vi "CalSumv.vi"(0 "AD1":u64, 1 "AD2":u64, 2 "REAL1":dbl, 3 "REAL2":dbl, 5 "InOrOut":u16(ring) items=["InSumv"=2, "OutSumv"=3], 8 "类型":u32(ring)=4 items=["PCI5121"=1, "PCI9810"=2, "USBCAN1"=3, "USBCAN2"=4, "PCI9820"=5, "CAN232"=6, "PCI5110"=7, "CANLite(mini)"=8, "ISA9620"=9, "ISA5420"=10, "PC104CAN"=11, "CANET"=17, "DNP9810"=13, "USBCAN-E-U"=20, "USBCAN-2E-U"=21], 10 "设备索引":u32(ring) items=["0", "1", "2", "3", "4", "5", "6", "7", "8", "9", "10", "11", "12", "13", "14", "15", ""], 12 "CAN路数":u32(ring) items=["0", "1"], 14 "ExternFlag":u8, 16 "ID Send":u32, 18 "DataLen":u8) -> (20 "发送状态":bool, 21 "Gain":dbl, 22 "Offset":i32 format="%x")   [LabVIEW 2013]
uses:
  BHN01/AutoBurn/Settings/ControlCAN.dll
panel:
  in  "设备索引 2":u32(ring) items=["0", "1", "2", "3", "4", "5", "6", "7", "8", "9", "10", "11", "12", "13", "14", "15", ""]
  in  "CAN路数 2":u32(ring) items=["0", "1"]
  in  "类型 2":u32(ring)=4 items=["PCI5121"=1, "PCI9810"=2, "USBCAN1"=3, "USBCAN2"=4, "PCI9820"=5, "CAN232"=6, "PCI5110"=7, "CANLite(mini)"=8, "ISA9620"=9, "ISA5420"=10, "PC104CAN"=11, "CANET"=17, "DNP9810"=13, "USBCAN-E-U"=20, "USBCAN-2E-U"=21]
  out "VCI_CAN_OBJ_T":T1 {"ID" format="%x"}
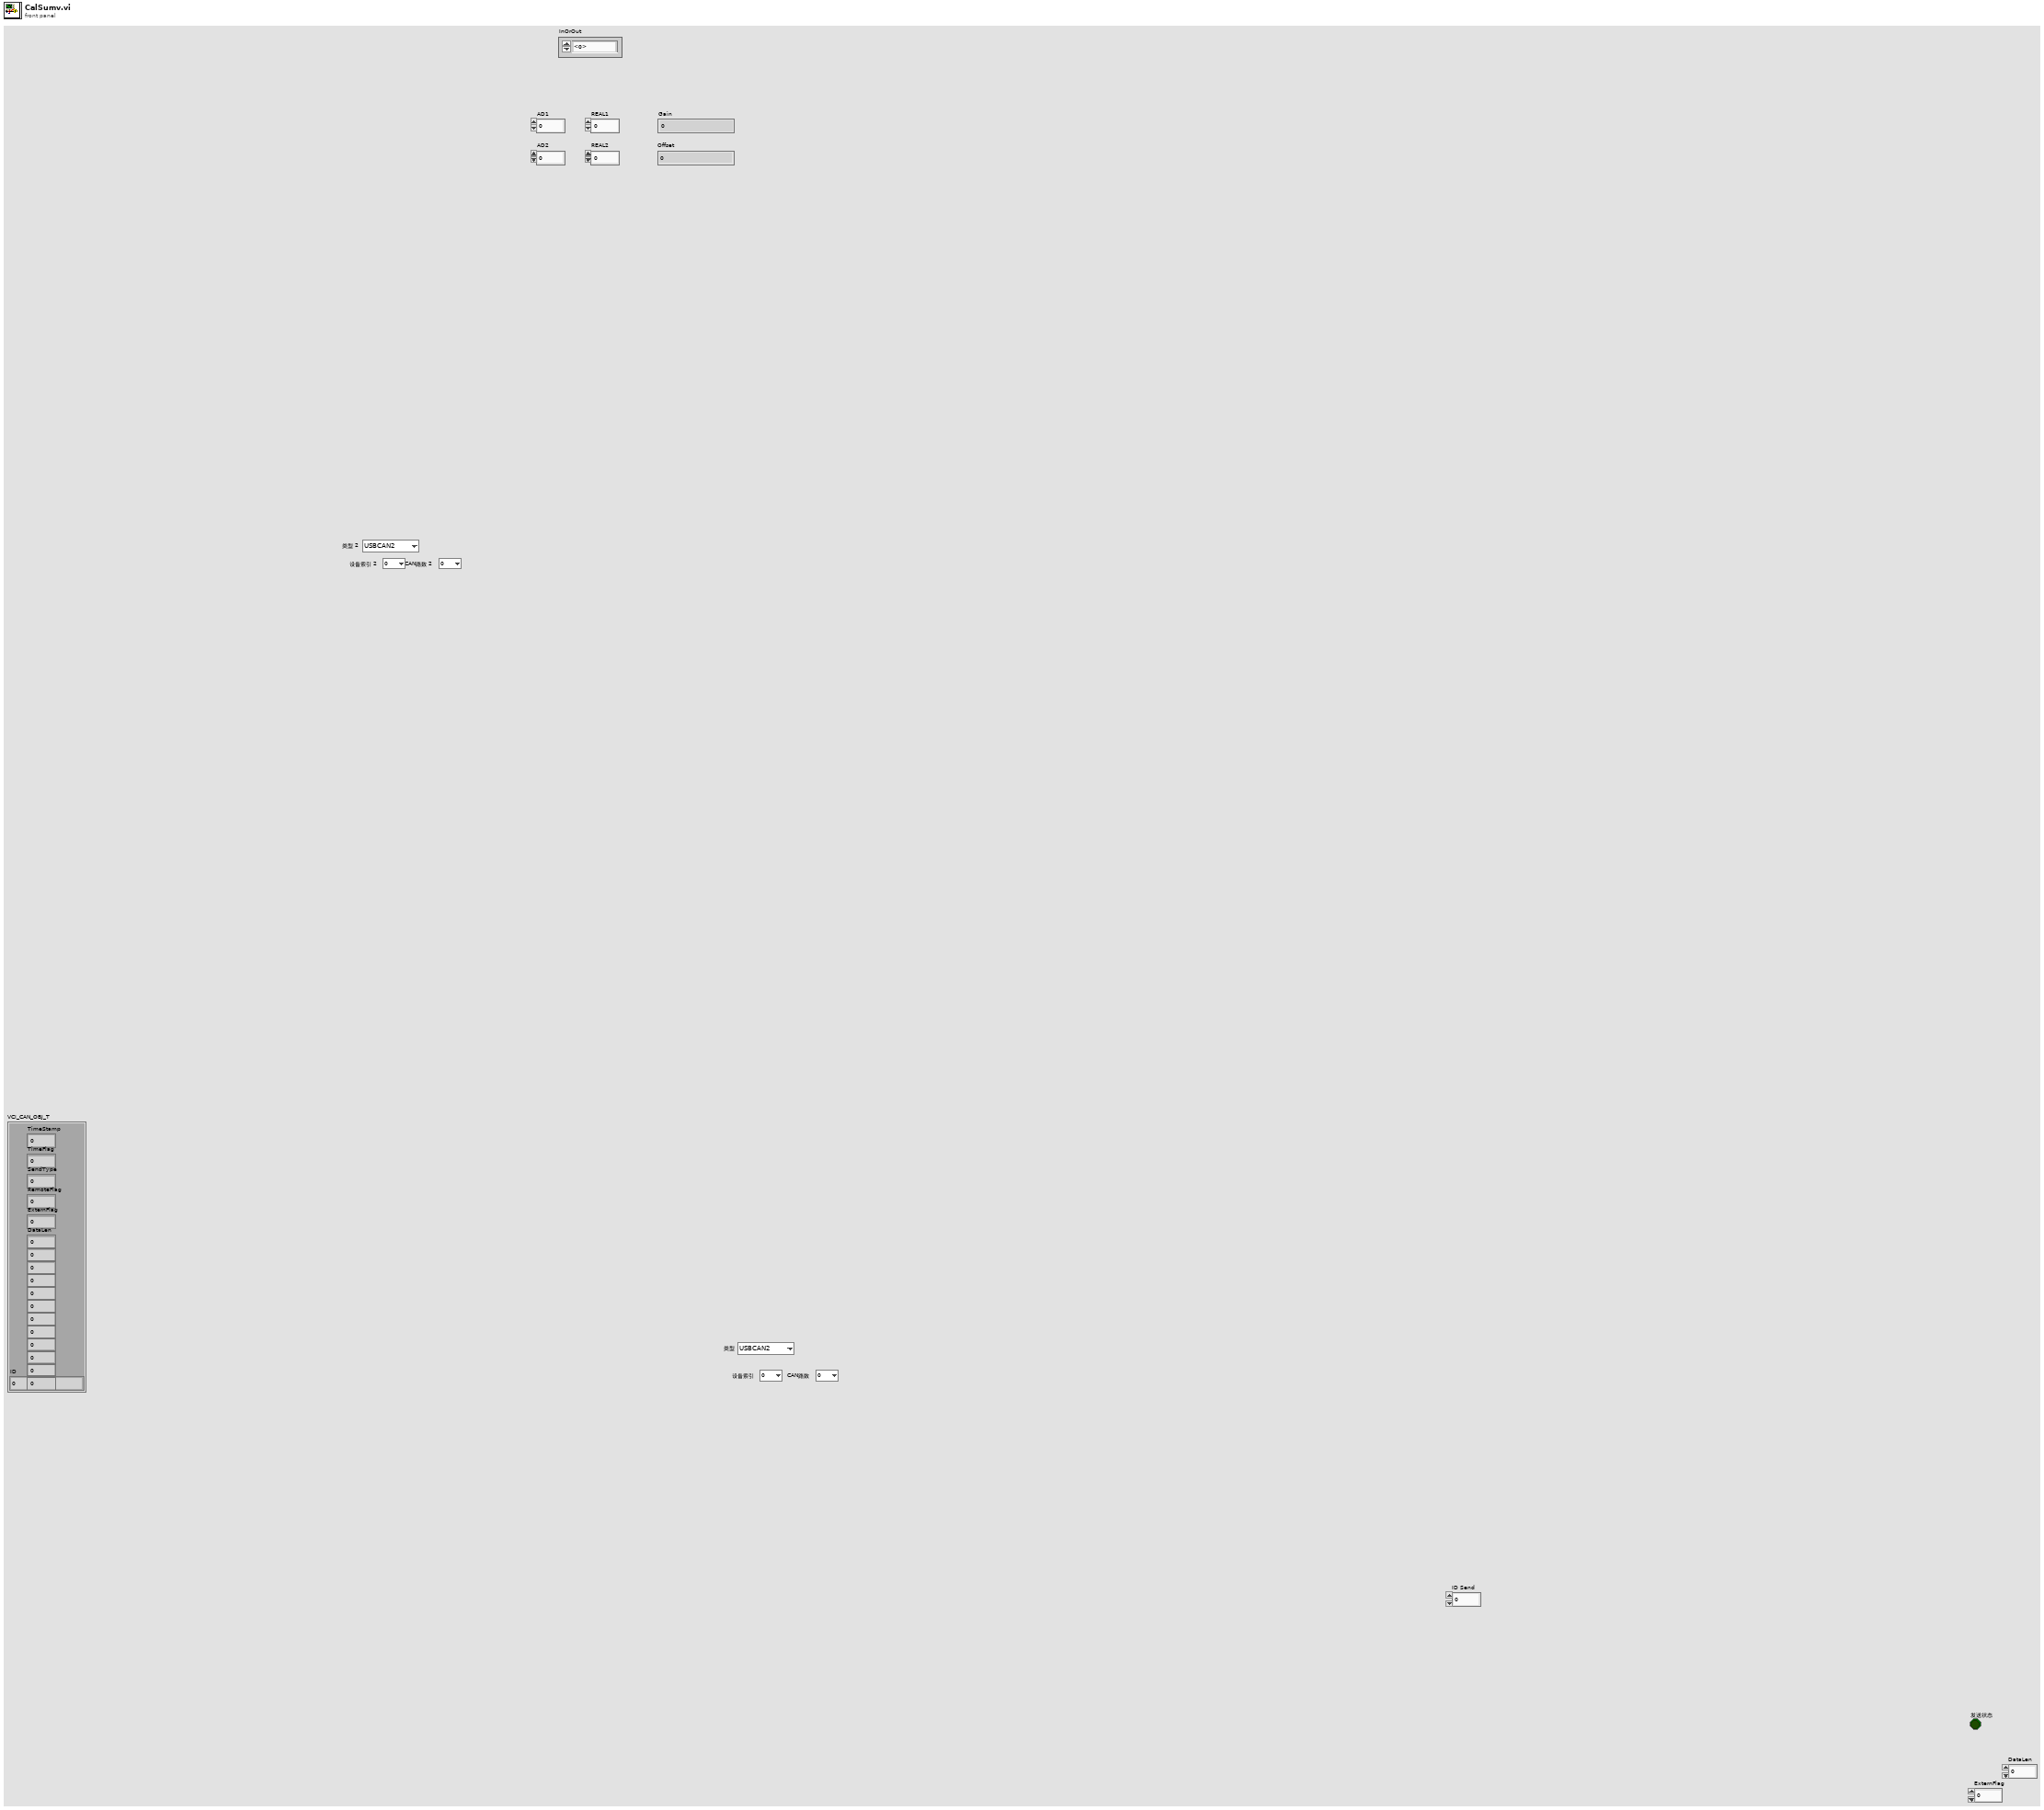
[diagram p1: front panel]
types:
  T1 = cluster{"ID":u32, "TimeStamp":u32, "TimeFlag":u8, "SendType":u8, "RemoteFlag":u8, "ExternFlag":u8, "DataLen":u8, u8, u8, u8, u8, u8, u8, u8, u8, u8, u8, u8}
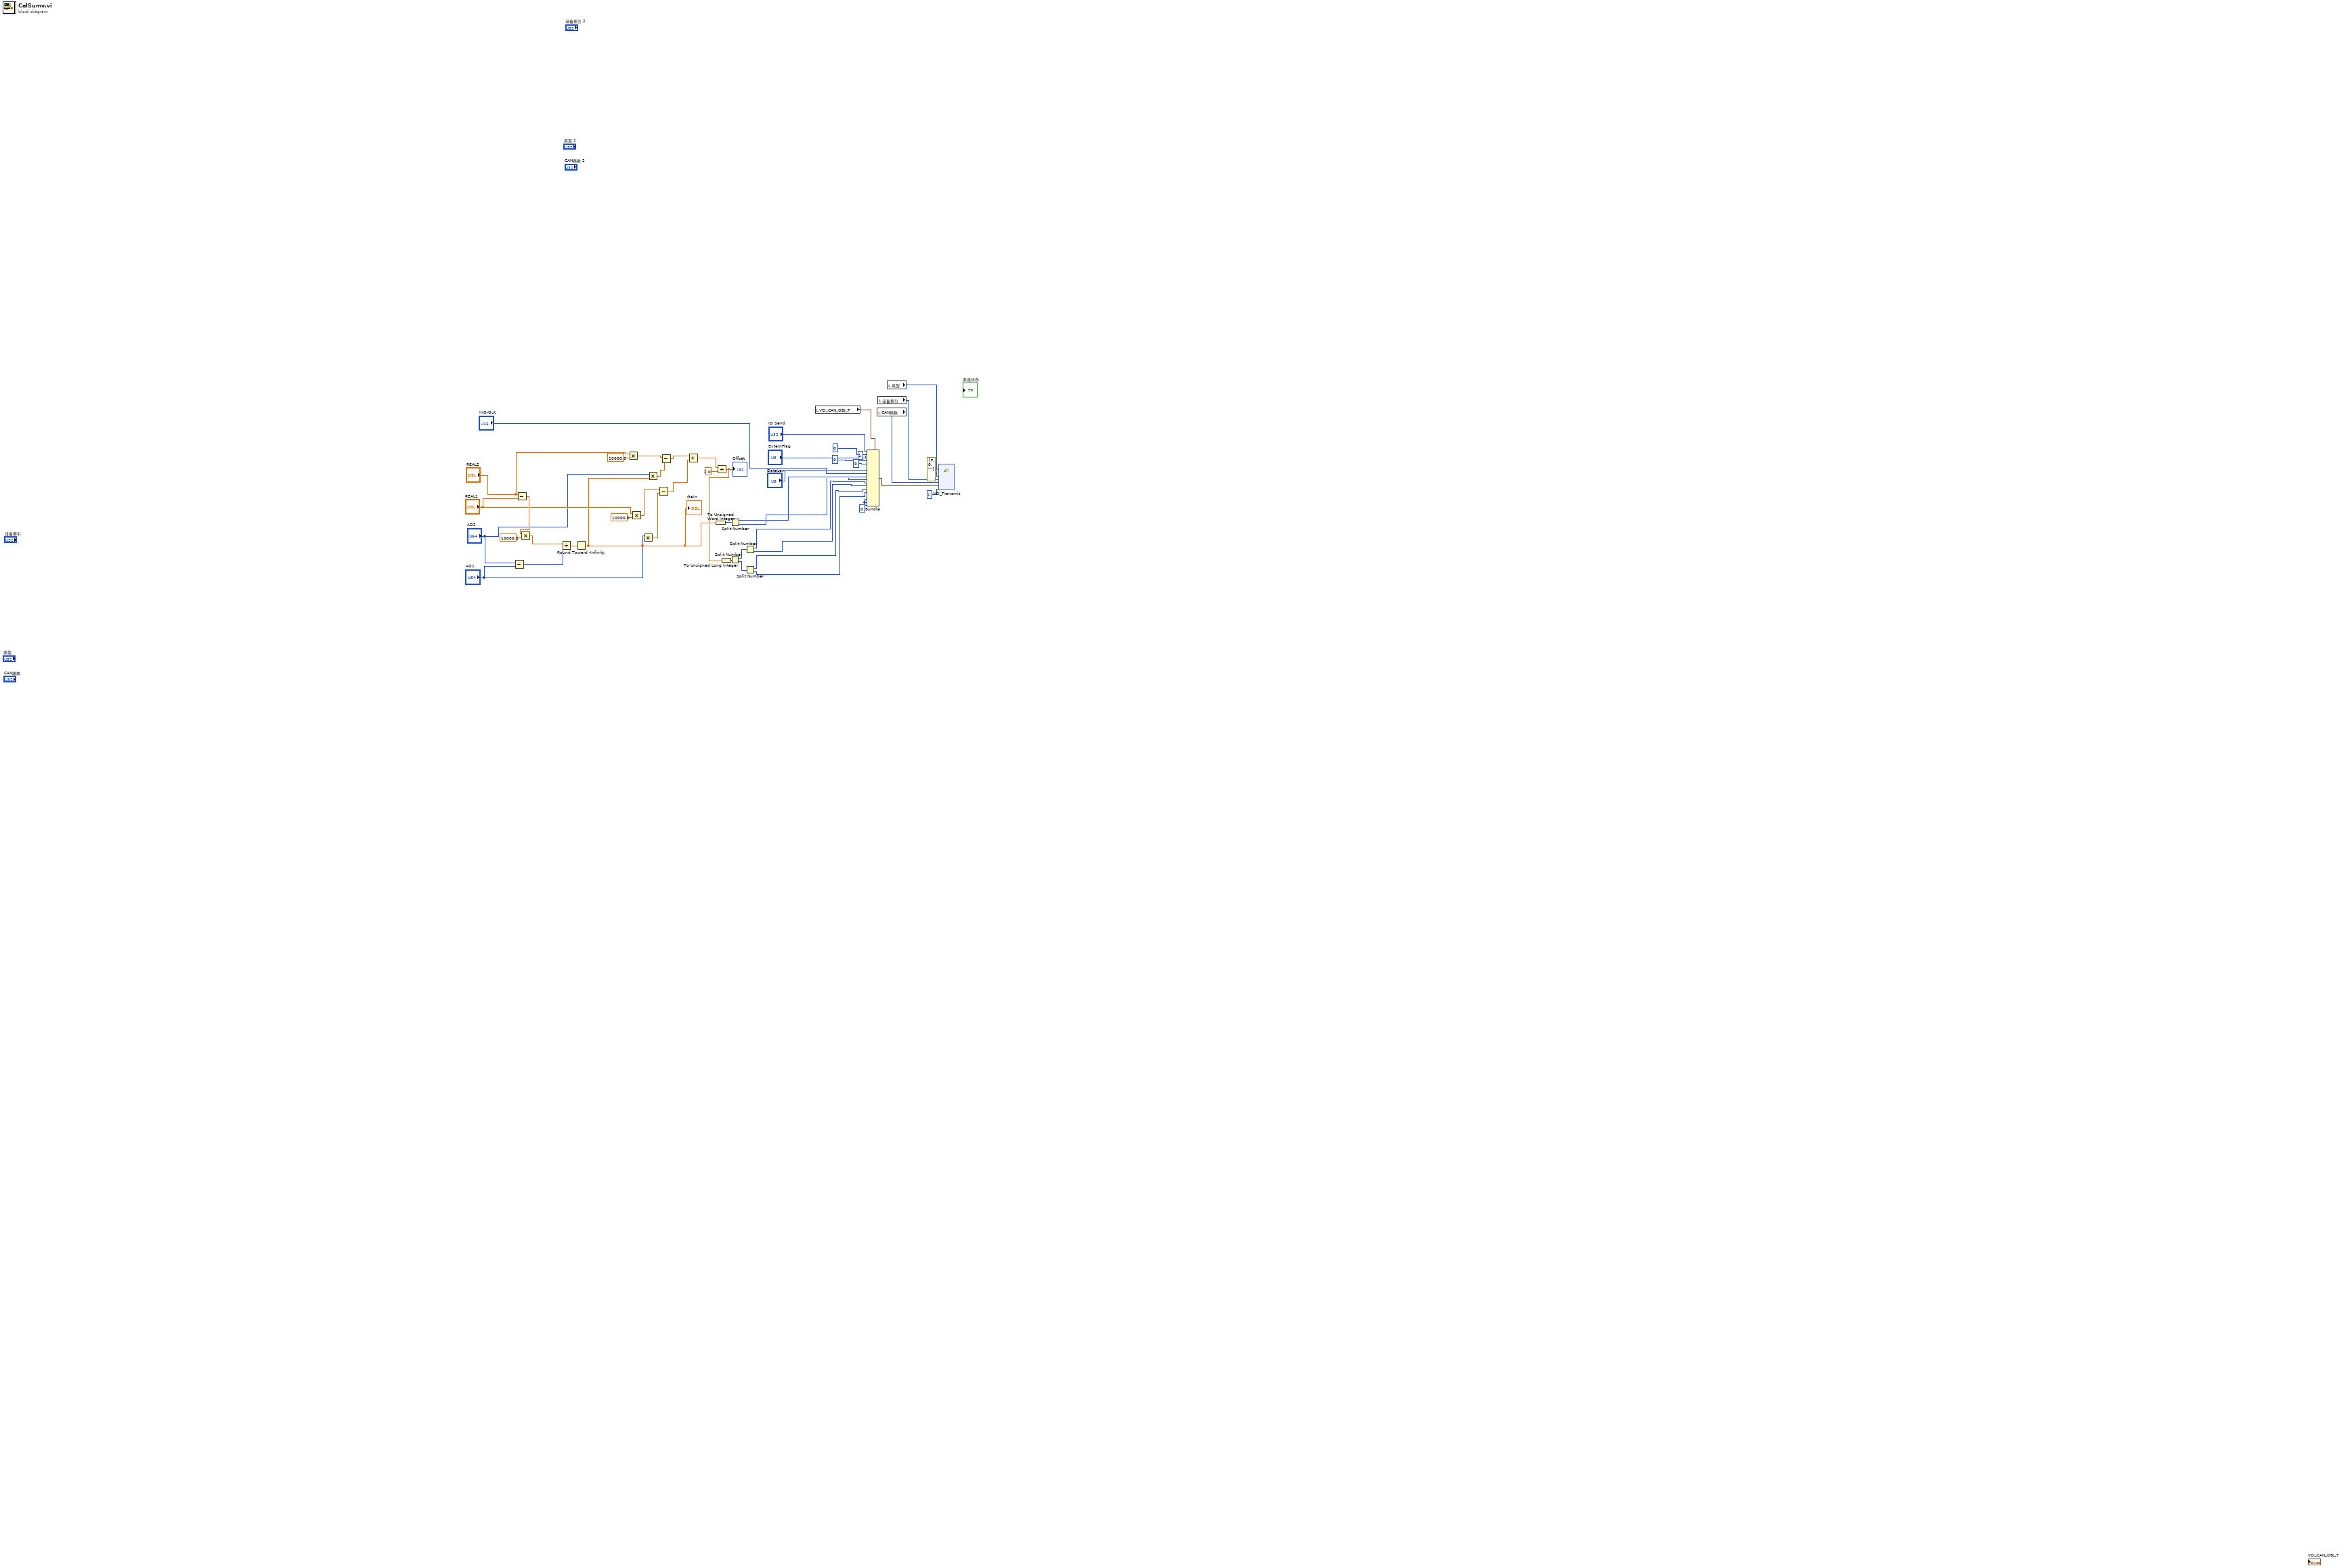
[diagram p0: block diagram]
diagram:
  w41 = u8 0 ("元素")
  n1 = Subtract(x="AD2", y="AD1") -> (x-y=w20:u64)
  n2 = Subtract(x="REAL2", y="REAL1") -> (x-y=w31:dbl)
  n3 = Multiply(x=w31, y=10000.0) -> (x*y=w30:dbl)
  n4 = Divide(x=w30, y=w20) -> (x/y=w14:dbl)
  n5 = Round Toward -Infinity(1:w14) -> (0:w13:dbl)
  "Gain" <- w13
  n6 = Multiply(x="REAL2", y=10000.0) -> (x*y=w22:dbl)
  n7 = Multiply(x="REAL1", y=10000.0) -> (x*y=w27:dbl)
  n8 = Multiply(x="AD1", y=w13) -> (x*y=w25:dbl)
  n9 = Multiply(x="AD2", y=w13) -> (x*y=w21:dbl)
  n10 = Subtract(x=w27, y=w25) -> (x-y=w18:dbl)
  n11 = Subtract(x=w22, y=w21) -> (x-y=w19:dbl)
  n12 = Add(x=w19, y=w18) -> (x+y=w17:dbl)
  n13 = To Unsigned Word Integer(number=w13) -> (unsigned 16bit integer=w12:u16)
  n14 = Divide(x=w17, y=2.0) -> (x/y=w11:dbl)
  "Offset" <- w11
  n15 = To Unsigned Long Integer(number=w11) -> (unsigned 32bit integer=w10:u32)
  n16 = Split Number(x=w10) -> (hi(x)=w9:u16, lo(x)=w8:u16)
  n17 = Split Number(x=w12) -> (hi(x)=w7:u8, lo(x)=w6:u8)
  n18 = Split Number(x=w9) -> (hi(x)=w5:u8, lo(x)=w4:u8)
  n19 = Split Number(x=w8) -> (hi(x)=w3:u8, lo(x)=w2:u8)
  n20 = local read "VCI_CAN_OBJ_T"() -> (w45:T1)
  n21 = Bundle(cluster=w45, "ID"="ID Send", "TimeStamp"=u8 0 ("RemoteFlag"), "TimeFlag"=u8 1, "SendType"=u8 0 ("DataLen"), "RemoteFlag"=u8 0, "ExternFlag"="ExternFlag", "DataLen"="DataLen", "InOrOut", w7, w6, w5, w4, w3, w2, w41, w41, w41) -> (w46:T1)  [unwired: 1 in]
  n22 = local read "CAN路数"() -> (w33:u32)
  n23 = local read "设备索引"() -> (w34:u32)
  n24 = local read "类型"() -> (w35:u32)
  n25 = dll-call lib="F:/Bluewave New Energy/SVN_Work/AutoTest_TestStand/trunk/AutoTest_TestStand/Driver/ZlgCan/BHN01/AutoBurn/Settings/ControlCAN.dll" fn="VCI_Transmit"(error in=errorcluster {"status"=FALSE, "code"=0, "source"=""} ("错误输入（无错误）"), "DeviceType"=w35, "DeviceInd"=w34, "CANInd"=w33, "pSend"=w46, "Len"=u32 1) -> ()  [unwired: 4 in, 6 out]
